vi "Colour.vi"(9 "result":string, 11 "colourRef":refnum<vi>) -> (3 "colourRef 2":refnum<vi>)   [LabVIEW 2020]
uses:
  Global_Variable/Global.vi
panel:
  in  "result 2":string
  in  "黄灯":bool
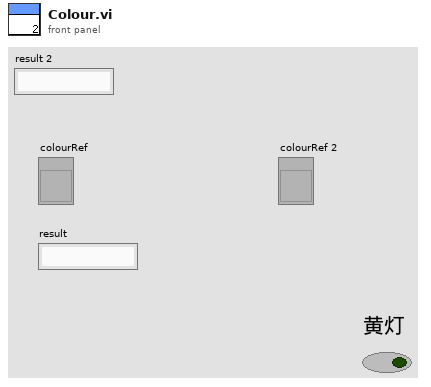
[diagram p1: front panel]
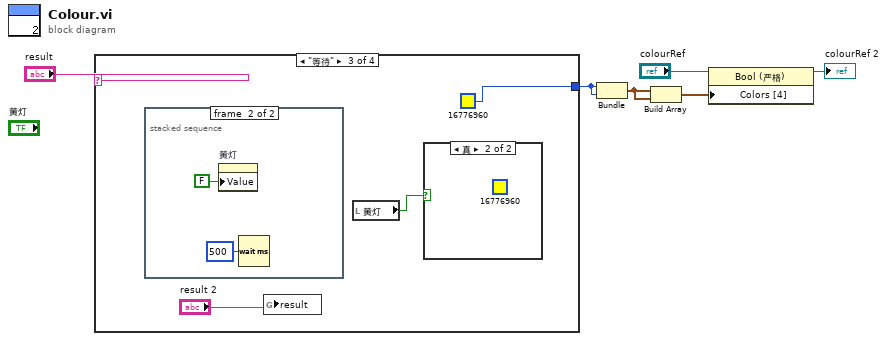
[diagram p0: block diagram]
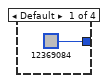
[diagram p2: hidden frame]
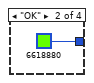
[diagram p3: hidden frame]
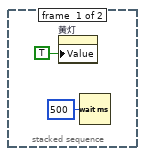
[diagram p5: hidden frame]
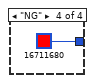
[diagram p6: hidden frame]
diagram:
  n1 = case shown="\"等待\"" "result" {
    tunnel: [u32 12369084 u32 6618880 u32 16776960 u32 16711680] -> w6
    frame Default {
    }
    frame "OK" {
    }
    frame "等待" {
      n2 = stacked-sequence {
        frame #0 {
          n3 = property on="黄灯" class="Bool (严格)"("Value"=TRUE ("黄灯")) -> ()  [unwired: 2 in, 2 out]
          n4 = Wait (ms)(milliseconds to wait=u32 500 ("等待时间（毫秒）")) -> ()  [unwired: 1 out]
        }
        frame #1 {
          n5 = property on="黄灯" class="Bool (严格)"("Value"=FALSE ("黄灯")) -> ()  [unwired: 2 in, 2 out]
          n6 = Wait (ms)(milliseconds to wait=u32 500 ("等待时间（毫秒）")) -> ()  [unwired: 1 out]
        }
      }
      n7 = global write "Global.vi" "result"("result 2") -> ()
      n8 = local read "黄灯"() -> (w11:bool)
      n9 = case shown="真" w11 {
        frame False {
        }
        frame True {
          (unwired) u32 16776960
        }
      }
    }
    frame "NG" {
    }
  }
  n10 = Bundle(w6, w6) -> (w5:cluster{u32, u32})  [unwired: 1 in]
  n11 = Build Array(w5, w5) -> (w1:cluster{u32, u32}[])
  n12 = property class="Bool (严格)"(reference="colourRef", "Colors [4]"=w1) -> (reference out=→"colourRef 2":refnum<vi>)  [unwired: 1 in, 1 out]
